vi "Dashboard Main.vi"() -> ()   [LabVIEW 2017]
uses:
  <vilib>/Utility/miscctls.llb/LVRowAndColumnTypeDef.ctl
  <vilib>/event_ctls.llb/eventvkey.ctl
  <vilib>/Rock Robotics/Network Tables/NT Read Numeric Array.vi
  <vilib>/Rock Robotics/WPI/Dashboard/WPI_DashboardLogging Global.vi
  <vilib>/Rock Robotics/Network Tables/NT Read Boolean.vi
panel:
  in  "Camera Settings Right":T1={"Frame Rate"=30, "Compression"=30, "Size"=1, "DB Camera Config"=FALSE} {"Frame Rate" scale=1.0..30.0; "Compression" scale=100.0..-1.0; "Size" items=["640x480", "320x240", "160x120"]}
  in  "Camera Name Right":string(combo)="No Camera Selection"
  out "Camera Info":cluster{"Mbps LED":bool, "Mbps":dbl, "fps":dbl} {"fps" format="%#.1g"; "Mbps" format="%#.1g"}
  in  "Camera Settings":T1={"Frame Rate"=30, "Compression"=30, "Size"=1, "DB Camera Config"=FALSE} {"Frame Rate" scale=1.0..30.0; "Compression" scale=100.0..-1.0; "Size" items=["640x480", "320x240", "160x120"]}
  in  "TCP":refnum<k5>
  in  "Rec Mode":enum32{"Stop", "Record", "Playback"}(radio)
  out "Robot IP":string
  out "Image Message":string="Timeout in Camera Communications"
  in  "Dashboard Tab":T2(tab)
  in  "Select Auto":string(combo)="Select Autonomous ..."
  out "NT Connection":bool
  out "MotorChart R":cluster{"Numeric":dbl, "Numeric":dbl}(graph)
  out "MotorChart L":cluster{"Numeric":dbl, "Numeric":dbl}(graph)
  out "MotorSliders R":cluster{"MotorSlide1":dbl, "MotorSlide2":dbl} {"MotorSlide2" scale=-1.0..1.0 scale format="%#_2e"; "MotorSlide1" scale=-1.0..1.0 scale format="%#_2e"}
  out "MotorSliders L":cluster{"MotorSlide1":dbl, "MotorSlide2":dbl} {"MotorSlide2" scale=-1.0..1.0 scale format="%#_2e"; "MotorSlide1" scale=-1.0..1.0 scale format="%#_2e"}
  out "Gyro":dbl(knob) scale=0.0..360.0
  out "JS1 Z":dbl(slide) scale=-1.0..1.0 scale format="%#_2e"
  out "JS1 Graph":cluster{"X":dbl, "Y":dbl}[](graph)
  out "JS1 Buttons":T3
  out "JS2 Z":dbl(slide) scale=-1.0..1.0 scale format="%#_2e"
  out "JS2 Graph":cluster{"X":dbl, "Y":dbl}[](graph)
  out "JS2 Buttons":T3
  out "Mode":T4(ring)=enum."Auto Disabled"
  out "Camera Image Right":T5(plugin-control)
  in  "DB/String 9":string
  in  "DB/String 8":string
  in  "DB/String 7":string
  in  "DB/String 6":string
  in  "DB/String 5":string
  in  "DB/String 4":string
  in  "DB/String 3":string
  in  "DB/String 2":string
  in  "DB/String 1":string
  in  "DB/String 0":string
  in  "DB/Slider 0":dbl(slide) scale=0.0..5.0
  in  "DB/Slider 1":dbl(slide) scale=0.0..5.0
  in  "DB/Slider 2":dbl(slide) scale=0.0..5.0
  in  "DB/Slider 3":dbl(slide) scale=0.0..5.0
  out "DB/LED 3":bool
  out "DB/LED 2":bool
  out "DB/LED 1":bool
  out "DB/LED 0":bool
  in  "DB/Button 3":bool
  in  "DB/Button 2":bool
  in  "DB/Button 1":bool
  in  "DB/Button 0":bool caption="New Name"
  in  "Test Slider":dbl(slide) scale=0.0..100.0 scale format="%#_3g"
  in  "On/Off":bool caption="Solenoid"
  in  "Test Name":u16(ring) items=["Select the test to run..."]
  in  "Test Tree":string(tree)
  in  "Motor":cluster{"Value":dbl, "Enable":bool} {"Value" scale=-1.0..1.0 scale format="%#_3g"}
  out "Progress":T6 {"Test Progress" scale=0.0..100.0}
  in  "Rev/Fwd":cluster{"Forward":bool, "Reverse":bool}
  in  "Test Ring":u16(ring) items=["Monochrome", "Color"]
  out "Cmd Status":string
  in  "Execute Command":bool
  in  "Command Params":string[][](table)
  in  "Command Selection":i32(listbox)
  in  "CheckList":i32(listbox)
  out "Tree":string(tree)
  out "Camera Image":T5(plugin-control)
  out "Background":bool
  in  "Camera Name":string(combo)="No Camera Selection"
  # "HW"
  # "HW"
  # "Joysticks"
  # "Drive Motors"
  # "Front"
  # "Right"
  # "Left"
  # "Back"
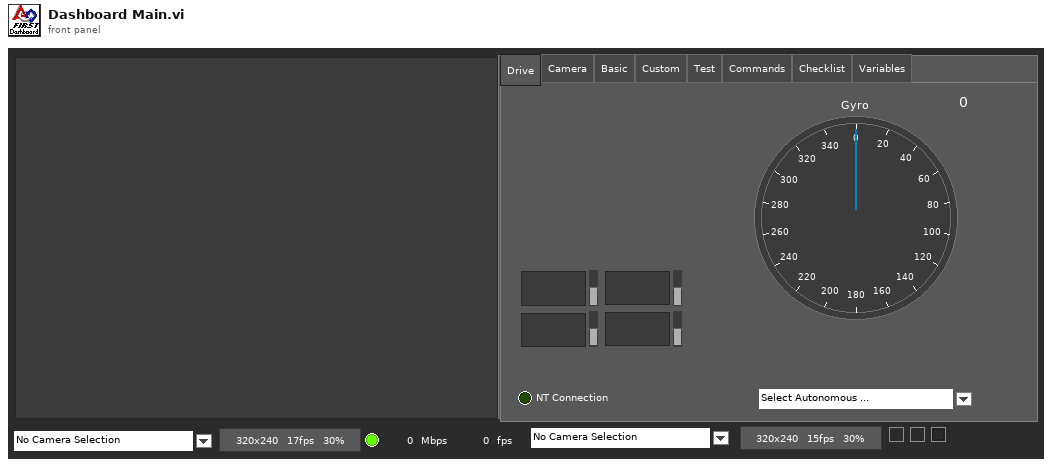
[diagram p1: front panel]
types:
  T1 = cluster{"Frame Rate":i32, "Compression":i32, "Size":u16, "DB Camera Config":bool}
  T2 = enum32{"Drive", "Camera", "Basic", "Custom", "Test", "Commands", "Checklist", "Variables"}
  T3 = cluster{bool, bool, bool, bool, bool, bool, bool, bool, bool, bool, bool, bool}
  T4 = enum8{"Tele-Op Disabled", "Tele-Op Enabled", "Auto Disabled", "Auto Enabled", "Test Disabled", "Test Enabled", "Disconnected", "No Code", "E-Stop"}
  T5 = typedef "IMAQ Image.ctl" = refnum<image>
  T6 = cluster{"Test Progress":u8, "Test Progress Text":string}
  T7 = cluster{"Save Path":path, "Interval (s)":dbl, "Keep":i32}
  T8 = typedef "Image Type" = u32
  T9 = cluster{"IDs":cluster{"RPC field ID":u16, "Unique ID":u16}, "String":string}
  T10 = cluster{"String":string, string, "Saved DB Images Info":cluster{"Save Path":path, "Interval (s)":dbl, "Keep":i32}}
  T11 = cluster{"Camera Image":refnum<vi>, "Dashboard Tab":refnum<vi>, "Background":refnum<vi>, "Rec Mode":refnum<vi>, "Test Slider":refnum<vi>, "On/Off ":refnum<vi>, "Test Ring":refnum<vi>, "Rev/Fwd":refnum<vi>, "Test Name":refnum<vi>, "Motor":refnum<vi>, "Progress":refnum<vi>, "CheckList":refnum<vi>, "Tree":refnum<vi>, "Test Tree":refnum<vi>, "Command Params":refnum<vi>, "Command Selection":refnum<vi>, "Execute Command":refnum<vi>, "Cmd Status":refnum<vi>, "Camera Settings":refnum<vi>, "Camera Name":refnum<vi>, "Camera Info":refnum<vi>, "Camera Settings Right":refnum<vi>, "Camera Name Right":refnum<vi>, "Camera Image Right":refnum<vi>}
  T12 = cluster{"Error Strings":string, "Disable Counts":cluster{u16, u16}, "Rail Faults":cluster{u16, u16, u16}, "Robot IP":string, "DB Mode":u8, "Event Info":cluster{"Name":string, "Type":u8, "Number":u16, "Replay":u8}}
  T13 = cluster{"Storage":cluster{"Disk Free":u64, "RAM Block":u32, "RAM free":u32}, "CPU Utilization":cluster{"CPU % ISR":sgl, "CPU % Time Crit":sgl, "CPU % Timed Str":sgl, "CPU % High":sgl, "CPU % Above":sgl, "CPU % Normal":sgl, "CPU % Low":sgl}, "CAN":cluster{"% Bus Utilization":sgl, "Bus Off Cnt":u32, "TX_FIFO Full Cnt":u32, "Receive Error Cnt":u8, "Transmit Error Cnt":u8}, "HID":cluster{"HID Outputs":u32, "Rumble Low":u16, "Rumble High":u16}[]}
  T14 = cluster{"Status bits":cluster{"Test Mode":bool, "Autonomous":bool, "Enabled":bool, "Code Start":bool, "Brownout":bool, "Reserved 2":bool, "Reserved 3":bool, "E-Stop":bool}, "Code Trace":cluster{"Disabled":bool, "TeleOp":bool, "Auto":bool, "Test":bool}, "Controller Type":enum16{"unknown", "cRIO", "roboRio"}, "Code?":enum16{"unknown", "noCode", "code"}, "Battery V":dbl}
  T15 = cluster{"Control Bits":cluster{"TestMode":bool, "Autonomous":bool, "Enabled":bool, "FMS Present":bool, bool, bool, bool, "E-Stop":bool}, "Team Station ":u8, "Countdown":sgl, "Joystick Values":cluster{"Axes":dbl[], "Buttons":bool[], "POVs":i16[]}[]}
  T16 = cluster{"Axes":dbl[], "Buttons":bool[], "POVs":i16[]}[]
  T17 = cluster{"Axes":dbl[], "Buttons":bool[], "POVs":i16[]}
  T18 = cluster{"Buttons[0]":bool, "Buttons[1]":bool, "Buttons[2]":bool, "Buttons[3]":bool, "Buttons[4]":bool, "Buttons[5]":bool, "Buttons[6]":bool, "Buttons[7]":bool, "Buttons[8]":bool, "Buttons[9]":bool, "Buttons[10]":bool, "Buttons[11]":bool}
  T19 = cluster{"Operation":enum16{"Update", "Clear"}, "Color Box":u32}[]
  T20 = typedef "eventvkey.ctl" = enum16{"ASCII", "Enter", "Return", "Shift", "Ctrl", "Alt", "Cmd", "Opt", "Caps", "NumLock", "Clear", "Break", "Up", "Down", "Left", "Right", "Insert", "Delete", "Home", "End", "PageUp", "PageDown", "Escape", "Help", "Pause", "ScrollLock", "F1", "F2", "F3", "F4", "F5", "F6", "F7", "F8", "F9", "F10", "F11", "F12", "F13", "F14", "F15", "F16", "F17", "F18", "F19", "F20", "F21", "F22", "F23", "F24", "Play", "VolumeUp", "VolumeDown", "Mute", "Two Byte Char"}
  T21 = cluster{"Image Size":bool, "Image Type":bool, "Pixel Value":bool, "ROI Information":bool, "Zoom Factor":bool}
  T22 = cluster{"Operation":enum16{"Update", "Clear"}, "Color Box":u32}
  T23 = typedef "LVRowAndColumnTypeDef.ctl" = cluster{"Row":i32, "Column":i32}
  T24 = cluster{"Shift":bool, "Ctrl":bool, "Alt":bool, "Cmd":bool, "Opt":bool}
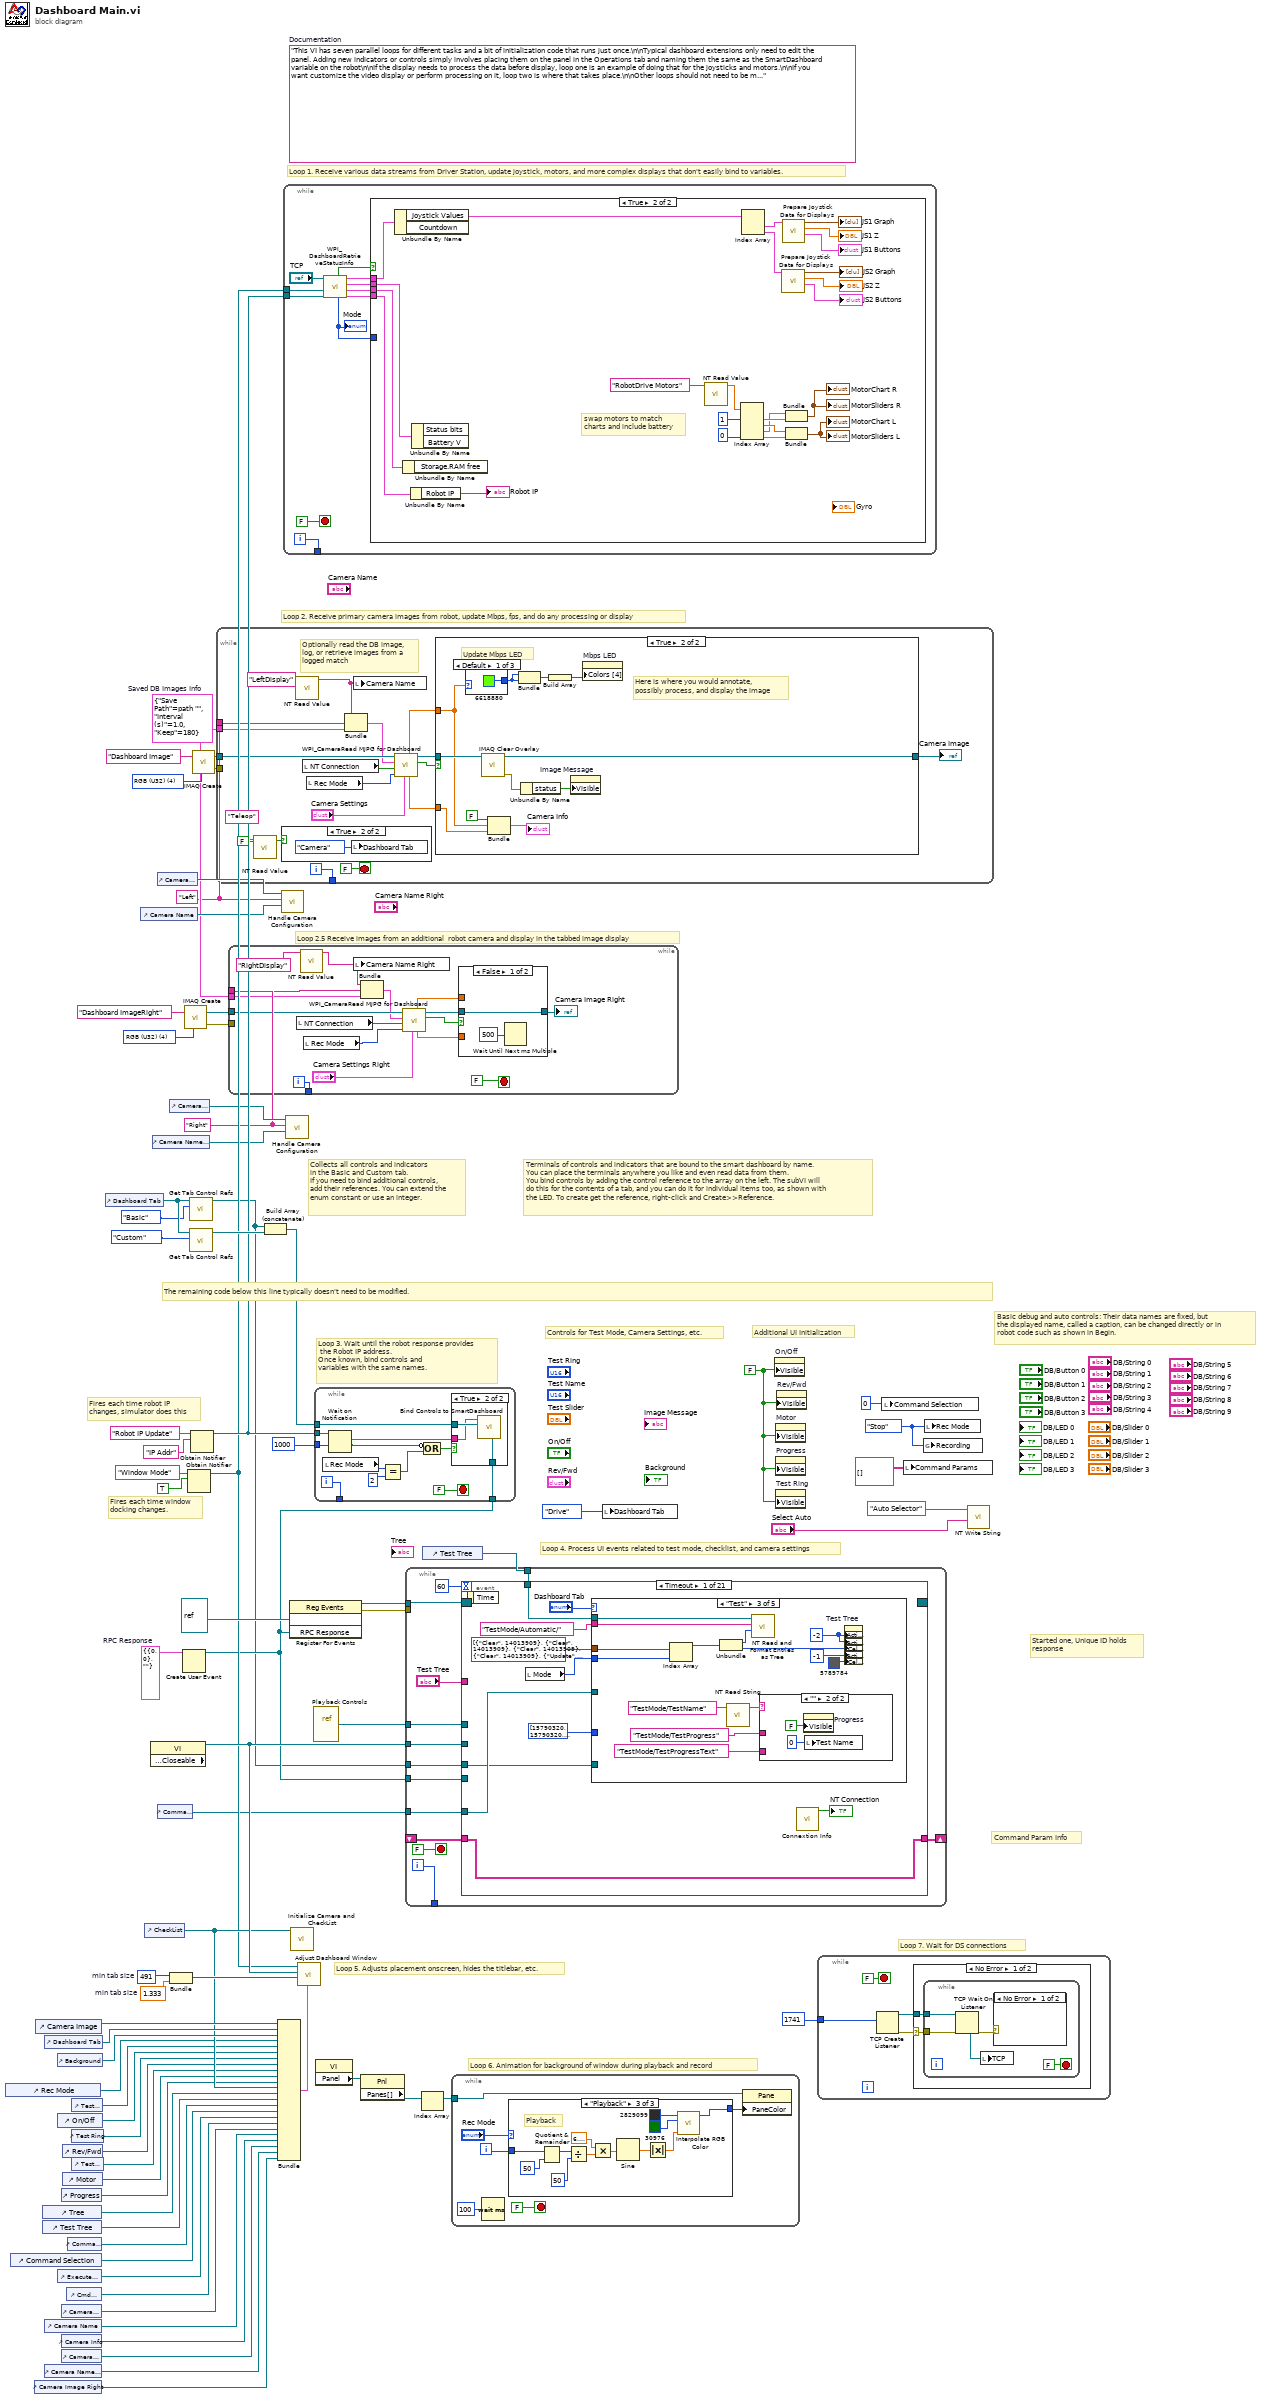
[diagram p0: block diagram]
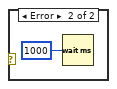
[diagram p3: hidden frame]
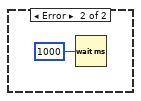
[diagram p4: hidden frame]
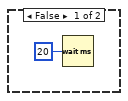
[diagram p5: hidden frame]
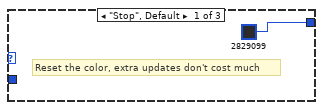
[diagram p6: hidden frame]
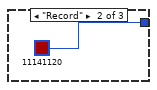
[diagram p7: hidden frame]
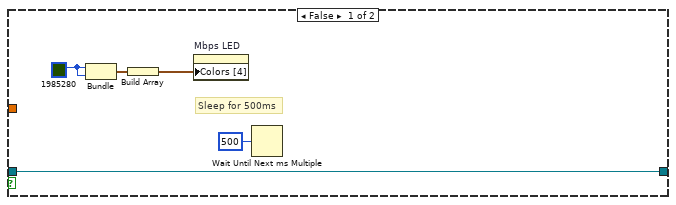
[diagram p10: hidden frame]
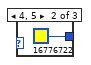
[diagram p11: hidden frame]
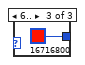
[diagram p12: hidden frame]
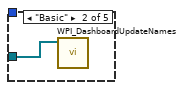
[diagram p14: hidden frame]
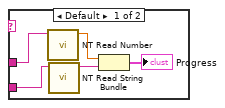
[diagram p15: hidden frame]
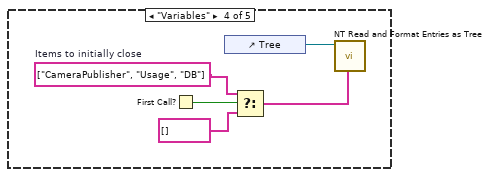
[diagram p16: hidden frame]
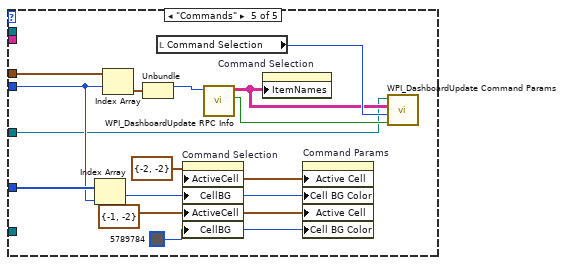
[diagram p17: hidden frame]
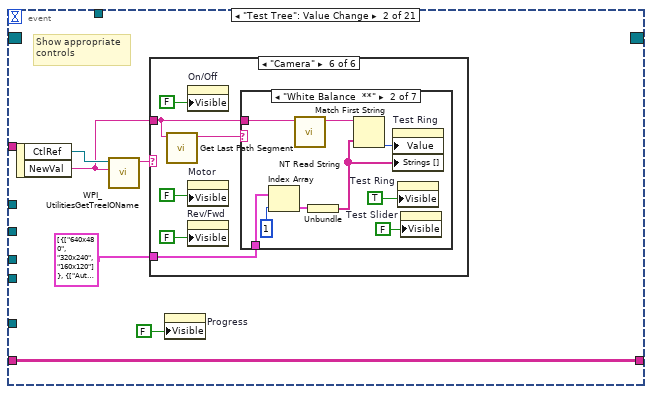
[diagram p18: hidden frame]
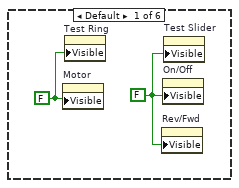
[diagram p19: hidden frame]
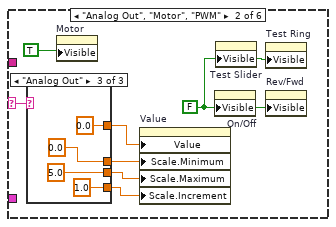
[diagram p20: hidden frame]
diagram:
  w3 = T7 {"Save Path"=path "", "Interval (s)"=1.0, "Keep"=180}  # Saved DB Images Info
  w2 = "Right"
  w1 = "Left"
  w13 = T8 4 items=["Grayscale (U8)", "Grayscale (I16)", "Grayscale (SGL)", "Complex (CSG)", "RGB (U32)", "HSL (U32)", "RGB (U64)"] ("Image Type")
  w29 = T9 {"IDs"={"RPC field ID"=0, "Unique ID"=0}, "String"=""}  # RPC Response
  w52 = 491  # min tab size
  w51 = 1.333  # min tab size
  w59 = enum32{"Stop", "Record", "Playback"}."Stop" ("Rec Mode")
  w36 = FALSE ("Visible")
  (unwired) "This VI has seven parallel loops for different tasks and a bit of initialization code that runs just once.\n\nTypical dashboard extensions only need to edit the panel. Adding new indicators or controls simply involves placing them on the panel in the Operations tab and naming them the same as the SmartDashboard variable on the robot\n\nIf the display needs to process the data before display, loop one is an example of doing that for the joysticks and motors.\n\nIf you want customize the video display or perform processing on it, loop two is where that takes place.\n\nOther loops should not need to be modified. They are pretty standard, and document the task they perform."  # Documentation
  w76 = T8 4 items=["Grayscale (U8)", "Grayscale (I16)", "Grayscale (SGL)", "Complex (CSG)", "RGB (U32)", "HSL (U32)", "RGB (U64)"] ("Image Type")
  # "Loop 2.5 Receive images from an additional  robot camera and display in the tabbed image display"
  # "Command Param Info"
  # "Started one, Unique ID holds\nresponse"
  # "Loop 7. Wait for DS connections"
  # "Basic debug and auto controls: Their data names are fixed, but\nthe displayed name, called a caption, can be changed directly or in\nrobot code such as shown in Begin."
  # "Controls for Test Mode, Camera Settings, etc."
  # "Additional UI Initialization"
  # "Loop 6. Animation for background of window during playback and record"
  # "Fires each time robot IP\nchanges, simulator does this"
  # "Fires each time window\ndocking changes."
  # "Collects all controls and indicators\nin the Basic and Custom tab.\nIf you need to bind additional controls,\nadd their references. You can extend the\nenum constant or use an integer."
  # "The remaining code below this line typically doesn't need to be modified."
  # "Loop 4. Process UI events related to test mode, checklist, and camera settings"
  # "Terminals of controls and indicators that are bound to the smart dashboard by name.\nYou can place the terminals anywhere you like and even read data from them.\nYou bind controls by adding the control reference to the array on the left. The subVI will\ndo this for the contents of a tab, and you can do it for individual items too, as shown with\nthe LED. To create get the reference, right-click and Create>>Reference."
  # "Loop 3. Wait until the robot response provides\n the Robot IP address.\nOnce known, bind controls and\nvariables with the same names."
  # "Loop 5. Adjusts placement onscreen, hides the titlebar, etc."
  # "Loop 1. Receive various data streams from Driver Station, update joystick, motors, and more complex displays that don't easily bind to variables."
  # "Loop 2. Receive primary camera images from robot, update Mbps, fps, and do any processing or display"
  n1 = control-ref of="Rec Mode"() -> (w42:refnum<vi>)
  n2 = control-ref of="Command Selection"() -> (w28:refnum<vi>)
  n3 = control-ref of="Camera Image Right"() -> (w6:refnum<vi>)
  n4 = control-ref of="Camera Image"() -> (w54:refnum<vi>)
  n5 = control-ref of="Tree"() -> (w46:refnum<vi>)
  n6 = control-ref of="Test Tree"() -> (w45:refnum<vi>)
  n7 = control-ref of="Dashboard Tab"() -> (w53:refnum<vi>)
  n8 = control-ref of="Camera Name"() -> (w19:refnum<vi>)
  n9 = control-ref of="Camera Name Right"() -> (w7:refnum<vi>)
  n10 = control-ref of="Execute Command"() -> (w30:refnum<vi>)
  n11 = control-ref of="Background"() -> (w49:refnum<vi>)
  n12 = control-ref of="On/Off"() -> (w40:refnum<vi>)
  n13 = control-ref of="Progress"() -> (w37:refnum<vi>)
  n14 = control-ref of="Camera Settings"() -> (w20:refnum<vi>)
  n15 = control-ref of="Camera Info"() -> (w18:refnum<vi>)
  n16 = control-ref of="Camera Settings Right"() -> (w8:refnum<vi>)
  n17 = control-ref of="Rev/Fwd"() -> (w38:refnum<vi>)
  n18 = control-ref of="Motor"() -> (w43:refnum<vi>)
  n19 = control-ref of="Cmd Status"() -> (w24:refnum<vi>)
  n20 = control-ref of="Command Params"() -> (w31:refnum<vi>)
  n21 = control-ref of="Test Slider"() -> (w41:refnum<vi>)
  n22 = control-ref of="Test Ring"() -> (w39:refnum<vi>)
  n23 = control-ref of="Test Name"() -> (w44:refnum<vi>)
  n24 = control-ref of="Dashboard Tab"() -> (w57:refnum<vi>)
  n25 = control-ref of="Camera Name"() -> (w21:refnum<vi>)
  n26 = control-ref of="CheckList"() -> (w47:refnum<vi>)
  n27 = property class="VI" props=["Front Panel.Closeable"]() -> (reference out=w58:refnum<vi>)  [unwired: 2 in, 2 out]
  n28 = control-ref of="Camera Name Right"() -> (w9:refnum<vi>)
  n29 = control-ref of="Camera Settings"() -> (w22:refnum<vi>)
  n30 = control-ref of="Command Params"() -> (w23:refnum<vi>)
  n31 = control-ref of="Camera Settings Right"() -> (w10:refnum<vi>)
  n32 = Bundle("min tab size"=w52, "min tab size"=w51) -> (w50:cluster{"min tab size":i32, "min tab size":dbl})  [unwired: 1 in]
  n33 = Create User Event(user event datatype=w29) -> (user event=w25:refnum<user-event>)  [unwired: 1 in, 1 out]
  n34 = call "IMAQ Create"("Image Name"="Dashboard ImageRight", "Image Type"=w13) -> ("New Image"=w12:T5, "error out"=w11:errorcluster)  [unwired: 2 in, 1 out]
  n35 = Obtain Notifier(name (unnamed)="Window Mode", notification data type=TRUE) -> (notifier out=w34:refnum<notifier>)  [unwired: 2 in, 2 out]
  n36 = call <vilib>:"Get Tab Control Refs.vi"("Page Index"=T2."Basic" ("Dashboard Tab"), "TabControl in"=w57) -> ("ControlsOnPage"=w17:refnum<vi>[])  [unwired: 9 in]
  n37 = call <vilib>:"Get Tab Control Refs.vi"("Page Index"=T2."Custom" ("Dashboard Tab"), "TabControl in"=w57) -> ("ControlsOnPage"=w56:refnum<vi>[])  [unwired: 9 in]
  n38 = Obtain Notifier(name (unnamed)="Robot IP Update", notification data type="IP Addr" ("name (unnamed)")) -> (notifier out=w35:refnum<notifier>)  [unwired: 2 in, 2 out]
  n39 = call "IMAQ Create"("Image Name"="Dashboard Image", "Image Type"=w76) -> ("New Image"=w74:T5, "error out"=w73:errorcluster)  [unwired: 2 in, 1 out]
  n40 = while {
    tunnel: w74 -> [w93]
    tunnel: w73 -> [_]
    tunnel: [w94] -> _
    tunnel: w3 -> [w84]
    tunnel: w1 -> [w82]
    i -> [w94]
    stop <- FALSE stop-if-true
    # "Optionally read the DB image,\nlog, or retrieve images from a\nlogged match"
    n41 = call-poly <vilib>:"NT Read Value.vi"("Default Value"=FALSE, "Name"="Teleop") -> ("Boolean"=w79:bool)  [unwired: 8 in, 1 out]
    n42 = case shown="True" w79 {
      frame False {
      }
      frame True {
        n43 = local write "Dashboard Tab"(T2."Camera" ("Dashboard Tab")) -> ()
      }
    }
    n44 = call-poly <vilib>:"NT Read Value.vi"("Name"="LeftDisplay") -> ("String"=w81:string)  [unwired: 9 in, 1 out]
    n45 = local read "NT Connection"() -> (w85:bool)
    n46 = local read "Rec Mode"() -> (w89:enum32{"Stop", "Record", "Playback"})
    n47 = Bundle("String"=w81, w82, "Saved DB Images Info"=w84) -> (w83:T10)  [unwired: 1 in]
    n48 = local write "Camera Name"(w81) -> ()
    n49 = call <vilib>:"WPI_CameraRead MJPG for Dashboard.vi"("Camera Settings"="Camera Settings", "Rec Mode"=w89, "NT Connection"=w85, "Capture Info"=w83, "Refnum in"=w93) -> ("Active"=w91:bool, "Refnum out"=w92:T5, "FPS"=w90:dbl, "Bandwidth (Mbps)"=w88:dbl)  [unwired: 3 in]
    n50 = case shown="True" w91 {
      tunnel: w92 -> [w97 w108]
      tunnel: w88 -> [_ w105]
      tunnel: w90 -> [_ w106]
      tunnel: [w97 w102] -> w86
      frame False {
        w99 = u32 1985280 ("Color Box")
        # "Sleep for 500ms"
        n51 = Bundle("Color Box"=w99, "Color Box"=w99) -> (w100:cluster{"Color Box":u32, "Color Box":u32})  [unwired: 1 out]
        n52 = Build Array(w100) -> (w98:cluster{"Color Box":u32, "Color Box":u32}[])
        n53 = property on="Mbps LED" class="Bool (strict)"("Colors [4]"=w98) -> ()  [unwired: 2 in, 2 out]
        n54 = Wait Until Next ms Multiple(millisecond multiple=u32 500) -> ()  [unwired: 1 out]
      }
      frame True {
        # "Here is where you would annotate,\npossibly process, and display the image"
        # "Update Mbps LED"
        n55 = case shown="Default" w105 {
          tunnel: [u32 6618880 ("Color Box") u32 16776722 ("Color Box") u32 16716800 ("Color Box")] -> w109
          frame Default {
          }
          frame 4, 5 {
          }
          frame 6.. {
          }
        }
        n56 = call "IMAQ Clear Overlay"("Image"=w108) -> ("error out"=w111:errorcluster, "Image Out"=w102:T5)  [unwired: 2 in, 7 out]
        n57 = Bundle(FALSE, "Bandwidth (Mbps)"=w105, "FPS"=w106) -> (→"Camera Info":cluster{bool, "Bandwidth (Mbps)":dbl, "FPS":dbl})  [unwired: 1 in]
        n58 = Bundle("Color Box"=w109, "Color Box"=w109) -> (w110:cluster{"Color Box":u32, "Color Box":u32})  [unwired: 1 out]
        n59 = Unbundle By Name(w111) -> ("status"=w112:bool)
        n60 = Build Array(w110) -> (w107:cluster{"Color Box":u32, "Color Box":u32}[])
        n61 = property on="Image Message" class="Str"("Visible"=w112) -> ()  [unwired: 2 in, 2 out]
        n62 = property on="Mbps LED" class="Bool (strict)"("Colors [4]"=w107) -> ()  [unwired: 2 in, 2 out]
      }
    }
    "Camera Image" <- w86
  }
  n63 = while {
    tunnel: w12 -> [w131]
    tunnel: w11 -> [_]
    tunnel: [w126] -> _
    tunnel: w3 -> [w120]
    tunnel: w2 -> [w119]
    i -> [w126]
    stop <- FALSE stop-if-true
    n64 = local read "NT Connection"() -> (w121:bool)
    n65 = call-poly <vilib>:"NT Read Value.vi"("Name"="RightDisplay") -> ("String"=w116:string)  [unwired: 9 in, 1 out]
    n66 = local read "Rec Mode"() -> (w130:enum32{"Stop", "Record", "Playback"})
    n67 = local write "Camera Name Right"(w116) -> ()
    n68 = Bundle("String"=w116, w119, "Saved DB Images Info"=w120) -> (w117:T10)  [unwired: 1 in]
    n69 = call <vilib>:"WPI_CameraRead MJPG for Dashboard.vi"("Camera Settings"="Camera Settings Right", "Rec Mode"=w130, "NT Connection"=w121, "Capture Info"=w117, "Refnum in"=w131) -> ("Active"=w125:bool, "Refnum out"=w128:T5, "FPS"=w123:dbl, "Bandwidth (Mbps)"=w124:dbl)  [unwired: 3 in]
    n70 = case shown="False" w125 {
      tunnel: w128 -> [w132 w134]
      tunnel: w124 -> [_ _]
      tunnel: w123 -> [_ _]
      tunnel: [w132 w134] -> w122
      frame False {
        n71 = Wait Until Next ms Multiple(millisecond multiple=u32 500) -> ()  [unwired: 1 out]
      }
      frame True {
      }
    }
    "Camera Image Right" <- w122
  }
  n72 = Build Array (concatenate)(w17, w56) -> (w55:refnum<vi>[])
  n73 = Bundle("Camera Image"=w54, "Dashboard Tab"=w53, "Background"=w49, "Rec Mode"=w42, "Test Slider"=w41, "On/Off"=w40, "Test Ring"=w39, "Rev/Fwd"=w38, "Test Name"=w44, "Motor"=w43, "Progress"=w37, "CheckList"=w47, "Tree"=w46, "Test Tree"=w45, "Command Params"=w31, "Command Selection"=w28, "Execute Command"=w30, "Cmd Status"=w24, "Camera Settings"=w20, "Camera Name"=w19, "Camera Info"=w18, "Camera Settings Right"=w8, "Camera Name Right"=w7, "Camera Image Right"=w6) -> (w48:T11)  [unwired: 1 in]
  n74 = call "Handle Camera Configuration.vi"("CameraNameRef"=w21, "Display Name"=w1, "ClusterRef"=w22) -> ()  [unwired: 9 in]
  n75 = while {
    tunnel: [w144] -> _
    tunnel: w35 -> [w138]
    tunnel: w34 -> [w135]
    i -> [w144]
    stop <- FALSE stop-if-true
    n76 = call <vilib>:"WPI_DashboardRetrieveStatusInfo.vi"("Binding Refnum"=w138, "Window Mode Notifier"=w135, "TCP Cnx"="TCP") -> ("Power and Errors"=w139:T12, "Robot Metrics"=w142:T13, "Status Info"=w143:T14, "Control Info"=w140:T15, "Robot Mode"=w137:T4, "Process?"=w141:bool)  [unwired: 3 in]
    "Mode" <- w137
    n77 = case shown="True" w141 {
      tunnel: w143 -> [_ w170]
      tunnel: w142 -> [_ w169]
      tunnel: w140 -> [_ w168]
      tunnel: w139 -> [_ w167]
      tunnel: w137 -> [_ _]
      frame False {
        n78 = Wait (ms)(milliseconds to wait=u32 20) -> ()  [unwired: 1 out]
      }
      frame True {
        # "swap motors to match\ncharts and include battery"
        n79 = Unbundle By Name(w168) -> ("Joystick Values"=w158:T16)  [unwired: 1 out]
        n80 = Unbundle By Name(w169) -> ()  [unwired: 1 out]
        n81 = Unbundle By Name(w167) -> ("Robot IP"=→"Robot IP":string)
        n82 = Unbundle By Name(w170) -> ()  [unwired: 2 out]
        n83 = call-poly <vilib>:"NT Read Value.vi"("Name"="RobotDrive Motors") -> ("Numeric Array"=w148:dbl[])  [unwired: 9 in, 1 out]
        n84 = Index Array(array=w148, index #1=1, index #4=0) -> (element #1=w162:dbl, element #2=w163:dbl, element #3=w161:dbl, element #4=w166:dbl)  [unwired: 2 in]
        n85 = Index Array(array=w158) -> (element #1=w157:T17, element #2=w153:T17)  [unwired: 2 in]
        n86 = call "Prepare Joystick Data for Displays.vi"("Joystick Values"=w153) -> ("Buttons"=→"JS2 Buttons":T18, "Z Axis"=→"JS2 Z":dbl, "Cartesian Data"=→"JS2 Graph":cluster{"X axis":dbl, "X axis":dbl}[])  [unwired: 8 in]
        n87 = call "Prepare Joystick Data for Displays.vi"("Joystick Values"=w157) -> ("Buttons"=→"JS1 Buttons":T18, "Z Axis"=→"JS1 Z":dbl, "Cartesian Data"=→"JS1 Graph":cluster{"X axis":dbl, "X axis":dbl}[])  [unwired: 8 in]
        n88 = Bundle("Numeric"=w161, "Numeric"=w162) -> (→"MotorChart R" →"MotorSliders R":cluster{"Numeric":dbl, "Numeric":dbl})  [unwired: 1 in]
        n89 = Bundle("Numeric"=w163, "Numeric"=w166) -> (→"MotorChart L" →"MotorSliders L":cluster{"Numeric":dbl, "Numeric":dbl})  [unwired: 1 in]
      }
    }
  }
  n90 = call "Handle Camera Configuration.vi"("CameraNameRef"=w9, "Display Name"=w2, "ClusterRef"=w10) -> ()  [unwired: 9 in]
  n91 = register-events(refnum<vi> refnum, w25) -> (reference out=w63:refnum<event-registration>, error out=w62:errorcluster)  [unwired: 2 in]
  n92 = call "Initialize Camera and CheckList.vi"("ListBox in"=w47) -> ()  [unwired: 11 in]
  n93 = call "Adjust Dashboard Window.vi"("Sizing Refnums"=w48, "Size Constraints"=w50, "VI"=w58, "WIn Mode"=w34) -> ()  [unwired: 8 in]
  n94 = vi-ref "Playback Controls.vi"() -> (w64:refnum<vi>)
  n95 = while {
    tunnel: w55 -> [w182]
    tunnel: w35 -> [w180]
    tunnel: [w178] -> _
    tunnel: u32 1000 ("milliseconds to wait") -> [w177]
    tunnel: w25 -> [w171]
    i -> [w178]
    stop <- FALSE stop-if-true
    n96 = local read "Rec Mode"() -> (w173:enum32{"Stop", "Record", "Playback"})
    n97 = Wait on Notification(notifier=w180, timeout in ms (-1)=w177) -> (notification=w179:string, timed out?=w175:bool)  [unwired: 2 in, 2 out]
    n98 = Equal?(x=w173, y=u16 2 ("Rec Mode")) -> (x = y?=w174:bool)
    n99 = Compound Arithmetic op=OR(invert w175, w174) -> (w176:bool)
    n100 = case shown="True" w176 {
      tunnel: w182 -> [_ w185]
      tunnel: w179 -> [_ w184]
      tunnel: w171 -> [_ w183]
      frame False {
      }
      frame True {
        n101 = call <vilib>:"Bind Controls to SmartDashboard.vi"("RPC ref"=w183, "Bound Control Refs"=w185, "Server IP Address"=w184) -> ()  [unwired: 9 in]
      }
    }
  }
  n102 = property class="VI"() -> ("Panel"=w66:refnum<vi>)  [unwired: 2 in, 2 out]
  n103 = property class="Pnl"(reference=w66) -> ("Panes[]"=w67:refnum<vi>[])  [unwired: 1 in, 2 out]
  n104 = Index Array(array=w67) -> (element=w65:refnum<vi>)  [unwired: 1 in]
  n105 = control-ref of="Test Tree"() -> (w68:refnum<vi>)
  n106 = while {
    tunnel: [w195] -> _
    tunnel: w68 -> [w194]
    tunnel: w64 -> [w193]
    tunnel: w63 -> [w192]
    tunnel: w62 -> [_]
    tunnel: w58 -> [w191]
    tunnel: w25 -> [w190]
    tunnel: w23 -> [w189]
    shift-right: [w188] -> _
    shift-left: _ -> [w187]
    tunnel: w17 -> [w186]
    i -> [w195]
    stop <- FALSE stop-if-true
    n107 = event shown="[0] Timeout" {
      selector: w192 -> [_ _ _ _ _ _ _ _ _ _ _ _ _ _ _ _ _ _ _ _ _]
      dyn-events: [_ _ _ _ _ _ _ _ _ _ _ _ _ _ _ _ w455 _ _ _ _] -> _
      timeout: u32 60 ("milliseconds to wait") -> [_ _ _ _ _ _ _ _ _ _ _ _ _ _ _ _ _ _ _ _ _]
      tunnel: w194 -> [w207 _ _ _ _ _ _ _ _ _ _ _ _ _ _ _ _ _ _ _ _]
      tunnel: "Test Tree" -> [_ _ _ _ _ _ _ _ _ _ _ w422 w430 w432 w436 w444 _ _ _ _ _]
      tunnel: w193 -> [_ _ _ _ _ _ _ _ _ _ _ _ _ _ _ _ w457 _ w475 _ _]
      tunnel: w191 -> [_ _ _ _ _ _ _ _ _ _ _ _ _ _ _ _ w453 _ _ _ _]
      tunnel: w190 -> [_ _ _ _ _ _ _ _ _ _ _ _ _ _ _ _ w451 _ _ _ _]
      tunnel: w189 -> [w202 _ _ _ _ _ w373 _ _ _ _ _ _ _ _ _ _ _ _ _ _]
      tunnel: [w201 w250 w352 w357 w366 w370 w371 w380 w390 w397 w409 w421 w428 w431 w435 w443 w450 w470 w472 w476 w489] -> w188
      tunnel: w187 -> [w201 w250 w352 w357 w366 w370 w371 _ _ w397 w409 w421 w428 w431 w435 w443 w450 w470 w472 w476 w489]
      tunnel: w186 -> [w199 _ _ _ _ _ _ _ _ _ _ _ _ _ _ _ _ _ _ _ _]
      event Timeout {
        n108 = event-data() -> ()  [unwired: 1 in, 1 out]
        n109 = local read "Mode"() -> (w204:T4)
        n110 = case shown="\"Test\"" "Dashboard Tab" {
          tunnel: w207 -> [_ _ w223 _ _]
          tunnel: "TestMode/Automatic/" ("Name Pattern") -> [_ _ w222 _ _]
          tunnel: T19 [{"Operation"=enum."Clear", "Color Box"=14013909}, {"Operation"=enum."Clear", "Color Box"=14013909}, {"Operation"=enum."Clear", "Color Box"=14013909}, {"Operation"=enum."Clear", "Color Box"=14013909}, {"Operation"=enum."Update", "Color Box"=14013909}, {"Operation"=enum."Update", "Color Box"=16777215}, {"Operation"=enum."Clear", "Color Box"=14013909}, {"Operation"=enum."Clear", "Color Box"=14013909}, {"Operation"=enum."Clear", "Color Box"=14013909}] -> [_ _ w215 _ w243]
          tunnel: w204 -> [_ _ w214 _ w242]
          tunnel: u32[] [15790320, 15790320, 15790320, 15790320, 16777215, 16777215, 15790320, 15790320, 15790320] -> [_ _ _ _ w248]
          tunnel: w202 -> [_ _ _ _ w236]
          tunnel: w199 -> [_ w209 _ _ _]
          frame "Custom", Default {
          }
          frame "Basic" {
            n111 = call <vilib>:"WPI_DashboardUpdateNames.vi"("Controls on Tab"=w209) -> ()  [unwired: 11 in]
          }
          frame "Test" {
            w221 = -2 ("Active Item:Row Number")
            n112 = Index Array(array=w215, index=w214) -> (element=w216:T22)
            n113 = Unbundle(w216) -> ("Operation"=w217:enum16{"Update", "Clear"}, "Color Box"=w218:u32)
            n114 = call <vilib>:"NT Read String.vi"("Name"="TestMode/TestName") -> ("String"=w212:string)  [unwired: 9 in, 1 out]
            n115 = call <vilib>:"NT Read and Format Entries as Tree.vi"("Operation"=w217, "Name Pattern"=w222, "Tree Refnum"=w223) -> ()  [unwired: 7 in, 2 out]
            n116 = case shown="\"\"" w212 {
              tunnel: "TestMode/TestProgress" ("Name") -> [w225 _]
              tunnel: "TestMode/TestProgressText" ("Name") -> [w224 _]
              frame Default {
                n117 = call <vilib>:"NT Read Number.vi"("Name"=w225) -> ("Numeric"=w226:dbl)  [unwired: 9 in, 1 out]
                n118 = call <vilib>:"NT Read String.vi"("Name"=w224) -> ("String"=w227:string)  [unwired: 9 in, 1 out]
                n119 = Bundle("Numeric"=w226, "String"=w227) -> (→"Progress":cluster{"Numeric":dbl, "String":string})  [unwired: 1 in]
              }
              frame "" {
                n120 = property on="Progress" class="Clust (strict)"("Visible"=FALSE) -> ()  [unwired: 2 in, 2 out]
                n121 = local write "Test Name"(u16 0) -> ()
              }
            }
            n122 = property on="Test Tree" class="Tree (strict)"("Active Item Row Number"=w221, "ActiveColNum"=w221, "CellBG"=w218, "Active Item Row Number"=-1 ("Active Item:Row Number"), "CellBG"=u32 5789784 ("Color Box")) -> ()  [unwired: 2 in, 2 out]
          }
          frame "Variables" {
            w233 = string[] ["CameraPublisher", "Usage", "DB"]  # Items to initially close
            n123 = First Call?() -> (First Call?: T/F=w234:bool)
            n124 = control-ref of="Tree"() -> (w235:refnum<vi>)
            n125 = Select(t=w233, s=w234, f=string[] []) -> (s? t:f=w231:string[])
            n126 = call <vilib>:"NT Read and Format Entries as Tree.vi"("Tags to  Close"=w231, "Tree Refnum"=w235) -> ()  [unwired: 8 in, 2 out]
          }
          frame "Commands" {
            w244 = u32 5789784 ("Color Box")
            w245 = T23 {"Row"=-1, "Column"=-2} ("Active Cell:Active Cell")
            w247 = T23 {"Row"=-2, "Column"=-2} ("Active Cell:Active Cell")
            n127 = Index Array(array=w248, index=w242) -> (element=w246:u32)
            n128 = Index Array(array=w243, index=w242) -> (element=w241:T22)
            n129 = Unbundle(w241) -> ("Operation"=w240:enum16{"Update", "Clear"})  [unwired: 1 out]
            n130 = local read "Command Selection"() -> (w239:i32)
            n131 = property on="Command Selection" class="MCListbox (strict)"("ActiveCell"=w247, "CellBG"=w246, "ActiveCell"=w245, "CellBG"=w244) -> ()  [unwired: 2 in, 2 out]
            n132 = call <vilib>:"WPI_DashboardUpdate RPC Info.vi"("Operation"=w240) -> ("update"=w238:bool, "commands"=w237:string[][])  [unwired: 9 in]
            n133 = property on="Command Selection" class="MCListbox (strict)"("ItemNames"=w237) -> ()  [unwired: 2 in, 2 out]
            n134 = property on="Command Params" class="Tbl (strict)"("Active Cell"=w247, "Cell BG Color"=w246, "Active Cell"=w245, "Cell BG Color"=w244) -> ()  [unwired: 2 in, 2 out]
            n135 = call <vilib>:"WPI_DashboardUpdate Command Params.vi"("Update"=w238, "NewVal"=w239, "Commands"=w237, "Param Tbl"=w236) -> ()  [unwired: 7 in, 1 out]
          }
        }
        n136 = call <vilib>:"Connextion Info.vi"() -> ("Connected"=→"NT Connection":bool)  [unwired: 10 in, 1 out]
      }
      event "Test Tree": Value Change {
        # "Show appropriate\ncontrols"
        n137 = event-data() -> ("CtlRef"=w253:refnum<vi>, "NewVal"=w251:string)  [unwired: 1 in]
        n138 = call <vilib>:"WPI_UtilitiesGetTreeIOName.vi"("NewVal"=w251, "TreeControl in"=w253) -> ("I/O Name"=w254:string)  [unwired: 9 in]
        n139 = case shown="\"Camera\"" w254 {
          selector: w254 -> [_ w261 _ w283 w292 _]
          tunnel: w251 -> [_ _ w280 w282 _ w299]
          tunnel: cluster{string[]}[] [{["640x480", "320x240", "160x120"]}, {["Auto", "Fixed indoor", "Fixed outdoor 1", "Fixed outdoor 2", "Fixed fluorescent 1", "Fixed fluorescent 2", "Hold current"]}, {["Auto", "Flicker-free 50 Hz", "Flicker-free 60 Hz", "Hold current"]}, {["None", "Prioritize frame rate", "Prioritize image quality"]}, {["Monochrome", "Color"]}] -> [_ _ _ _ _ w298]
          frame Default {
            w256 = FALSE ("Visible")
            w255 = FALSE ("Visible")
            n140 = property on="Motor" class="Clust (strict)"("Visible"=w255) -> ()  [unwired: 2 in, 2 out]
            n141 = property on="Test Ring" class="Ring (strict)"("Visible"=w255) -> ()  [unwired: 2 in, 2 out]
            n142 = property on="Rev/Fwd" class="Clust (strict)"("Visible"=w256) -> ()  [unwired: 2 in, 2 out]
            n143 = property on="On/Off" class="Bool (strict)"("Visible"=w256) -> ()  [unwired: 2 in, 2 out]
            n144 = property on="Test Slider" class="Slide (strict)"("Visible"=w256) -> ()  [unwired: 2 in, 2 out]
          }
          frame "Analog Out", "Motor", "PWM" {
            w262 = FALSE ("Visible")
            n145 = case shown="\"Analog Out\"" w261 {
              tunnel: [1.0 ("Value") -1.0 ("Value") 0.0 ("Value")] -> w260
              tunnel: [255.0 ("Value") 1.0 ("Value") 5.0 ("Value")] -> w259
              tunnel: [128.0 ("Value") 0.0 ("Value") 0.0 ("Value")] -> w258
              tunnel: [64.0 ("Value") 0.5 ("Value") 1.0 ("Value")] -> w257
              frame "PWM" {
              }
              frame "Motor", Default {
              }
              frame "Analog Out" {
              }
            }
            n146 = property on="Motor" class="Clust (strict)"("Visible"=TRUE) -> ()  [unwired: 2 in, 2 out]
            n147 = property on="Value" class="Slide (strict)"("Value"=w258, "Scale.Minimum"=w260, "Scale.Maximum"=w259, "Scale.Increment"=w257) -> ()  [unwired: 2 in, 2 out]
            n148 = property on="On/Off" class="Bool (strict)"("Visible"=w262) -> ()  [unwired: 2 in, 2 out]
            n149 = property on="Test Slider" class="Slide (strict)"("Visible"=w262) -> ()  [unwired: 2 in, 2 out]
            n150 = property on="Test Ring" class="Ring (strict)"("Visible"=w262) -> ()  [unwired: 2 in, 2 out]
            n151 = property on="Rev/Fwd" class="Clust (strict)"("Visible"=w262) -> ()  [unwired: 2 in, 2 out]
          }
          frame "Servo" {
            w278 = FALSE ("Visible")
            n152 = call <vilib>:"NT Read Number.vi"("Name"=w280) -> ("Numeric"=w279:dbl)  [unwired: 9 in, 1 out]
            n153 = property on="Test Slider" class="Slide (strict)"("Visible"=TRUE, "Scale.Maximum"=170.0 ("Scale.Range:Maximum")) -> ()  [unwired: 2 in, 2 out]
            n154 = local write "Test Slider"(w279) -> ()
            n155 = property on="Motor" class="Clust (strict)"("Visible"=w278) -> ()  [unwired: 2 in, 2 out]
            n156 = property on="Rev/Fwd" class="Clust (strict)"("Visible"=w278) -> ()  [unwired: 2 in, 2 out]
            n157 = property on="On/Off" class="Bool (strict)"("Visible"=w278) -> ()  [unwired: 2 in, 2 out]
            n158 = property on="Test Ring" class="Ring (strict)"("Visible"=w278) -> ()  [unwired: 2 in, 2 out]
          }
          frame "Relay", "Solenoid" {
            w281 = FALSE ("Visible")
            n159 = property on="Motor" class="Clust (strict)"("Visible"=w281) -> ()  [unwired: 2 in, 2 out]
            n160 = property on="Test Slider" class="Slide (strict)"("Visible"=w281) -> ()  [unwired: 2 in, 2 out]
            n161 = Search and Replace String(input string=w282, search string="/Value  **", replace string="/Direction") -> (result string=w288:string)  [unwired: 5 in, 3 out]
            n162 = property on="Test Ring" class="Ring (strict)"("Visible"=w281) -> ()  [unwired: 2 in, 2 out]
            n163 = call <vilib>:"NT Read String.vi"("Name"=w288) -> ("String"=w286:string)  [unwired: 9 in, 1 out]
            n164 = Equal?(x="Both directions", y=w286) -> (x = y?=w284:bool)
            n165 = Not(x=w284) -> (.not. x?=w285:bool)
            n166 = property on="Rev/Fwd" class="Clust (strict)"("Visible"=w284) -> ()  [unwired: 2 in, 2 out]
            n167 = property on="On/Off" class="Bool (strict)"("Visible"=w285, "Caption.Text"=w283) -> ()  [unwired: 2 in, 2 out]
          }
          frame "Compressor", "Digital Out" {
            w291 = FALSE ("Visible")
            # "Get direction and finish"
            n168 = property on="Motor" class="Clust (strict)"("Visible"=w291) -> ()  [unwired: 2 in, 2 out]
            n169 = property on="Test Slider" class="Slide (strict)"("Visible"=w291) -> ()  [unwired: 2 in, 2 out]
            n170 = property on="Test Ring" class="Ring (strict)"("Visible"=w291) -> ()  [unwired: 2 in, 2 out]
            n171 = property on="On/Off" class="Bool (strict)"("Visible"=TRUE, "Caption.Text"=w292) -> ()  [unwired: 2 in, 2 out]
            n172 = property on="Rev/Fwd" class="Clust (strict)"("Visible"=FALSE) -> ()  [unwired: 2 in, 2 out]
          }
          frame "Camera" {
            n173 = call <vilib>:"Get Last Path Segment.vi"("String in"=w299) -> ("String out"=w300:string)  [unwired: 10 in]
            n174 = property on="On/Off" class="Bool (strict)"("Visible"=FALSE) -> ()  [unwired: 2 in, 2 out]
            n175 = property on="Motor" class="Clust (strict)"("Visible"=FALSE) -> ()  [unwired: 2 in, 2 out]
            n176 = property on="Rev/Fwd" class="Clust (strict)"("Visible"=FALSE) -> ()  [unwired: 2 in, 2 out]
            n177 = case shown="\"White Balance  **\"" w300 {
              tunnel: w299 -> [w306 w315 w324 w333 w342 _ w348]
              tunnel: w298 -> [w304 w312 w321 w330 w339 _ _]
              frame "Size  **" {
                n178 = Index Array(array=w304) -> (element=w303:cluster{string[]})  [unwired: 1 in]
                n179 = call <vilib>:"NT Read String.vi"("Name"=w306) -> ("String"=w305:string)  [unwired: 9 in, 1 out]
                n180 = Unbundle(w303) -> (w301:string[])
                n181 = Match First String(2:w301, 3:w305) -> (0:w302:i32)  [unwired: 1 out]
                n182 = property on="Test Ring" class="Ring (strict)"("Value"=w302, "Strings []"=w301) -> ()  [unwired: 2 in, 2 out]
                n183 = property on="Test Ring" class="Ring (strict)"("Visible"=TRUE) -> ()  [unwired: 2 in, 2 out]
                n184 = property on="Test Slider" class="Slide (strict)"("Visible"=FALSE) -> ()  [unwired: 2 in, 2 out]
              }
              frame "White Balance  **" {
                n185 = Index Array(array=w312, index=1) -> (element=w313:cluster{string[]})
                n186 = call <vilib>:"NT Read String.vi"("Name"=w315) -> ("String"=w314:string)  [unwired: 9 in, 1 out]
                n187 = Unbundle(w313) -> (w310:string[])
                n188 = Match First String(2:w310, 3:w314) -> (0:w309:i32)  [unwired: 1 out]
                n189 = property on="Test Ring" class="Ring (strict)"("Value"=w309, "Strings []"=w310) -> ()  [unwired: 2 in, 2 out]
                n190 = property on="Test Ring" class="Ring (strict)"("Visible"=TRUE) -> ()  [unwired: 2 in, 2 out]
                n191 = property on="Test Slider" class="Slide (strict)"("Visible"=FALSE) -> ()  [unwired: 2 in, 2 out]
              }
              frame "Exposure  **" {
                n192 = Index Array(array=w321, index=2) -> (element=w322:cluster{string[]})
                n193 = call <vilib>:"NT Read String.vi"("Name"=w324) -> ("String"=w323:string)  [unwired: 9 in, 1 out]
                n194 = Unbundle(w322) -> (w318:string[])
                n195 = Match First String(2:w318, 3:w323) -> (0:w319:i32)  [unwired: 1 out]
                n196 = property on="Test Ring" class="Ring (strict)"("Value"=w319, "Strings []"=w318) -> ()  [unwired: 2 in, 2 out]
                n197 = property on="Test Ring" class="Ring (strict)"("Visible"=TRUE) -> ()  [unwired: 2 in, 2 out]
                n198 = property on="Test Slider" class="Slide (strict)"("Visible"=FALSE) -> ()  [unwired: 2 in, 2 out]
              }
              frame "Exposure Priority  **" {
                n199 = Index Array(array=w330, index=3) -> (element=w331:cluster{string[]})
                n200 = call <vilib>:"NT Read String.vi"("Name"=w333) -> ("String"=w332:string)  [unwired: 9 in, 1 out]
                n201 = Unbundle(w331) -> (w327:string[])
                n202 = Match First String(2:w327, 3:w332) -> (0:w328:i32)  [unwired: 1 out]
                n203 = property on="Test Ring" class="Ring (strict)"("Value"=w328, "Strings []"=w327) -> ()  [unwired: 2 in, 2 out]
                n204 = property on="Test Ring" class="Ring (strict)"("Visible"=TRUE) -> ()  [unwired: 2 in, 2 out]
                n205 = property on="Test Slider" class="Slide (strict)"("Visible"=FALSE) -> ()  [unwired: 2 in, 2 out]
              }
              frame "Color Enable  **" {
                n206 = Index Array(array=w339, index=4) -> (element=w340:cluster{string[]})
                n207 = call <vilib>:"NT Read String.vi"("Name"=w342) -> ("String"=w341:string)  [unwired: 9 in, 1 out]
                n208 = Unbundle(w340) -> (w336:string[])
                n209 = Match First String(2:w336, 3:w341) -> (0:w337:i32)  [unwired: 1 out]
                n210 = property on="Test Ring" class="Ring (strict)"("Value"=w337, "Strings []"=w336) -> ()  [unwired: 2 in, 2 out]
                n211 = property on="Test Ring" class="Ring (strict)"("Visible"=TRUE) -> ()  [unwired: 2 in, 2 out]
                n212 = property on="Test Slider" class="Slide (strict)"("Visible"=FALSE) -> ()  [unwired: 2 in, 2 out]
              }
              frame Default {
                n213 = property on="Test Ring" class="Ring (strict)"("Visible"=FALSE) -> ()  [unwired: 2 in, 2 out]
                n214 = property on="Test Slider" class="Slide (strict)"("Visible"=FALSE) -> ()  [unwired: 2 in, 2 out]
              }
              frame "Brightness  **", "Color Level  **", "Compression  **", "FPS  **", "Sharpness  **" {
                n215 = call <vilib>:"NT Read Number.vi"("Name"=w348) -> ("Numeric"=w347:dbl)  [unwired: 9 in, 1 out]
                n216 = local write "Test Slider"(w347) -> ()
                n217 = property on="Test Slider" class="Slide (strict)"("Visible"=TRUE, "Scale.Maximum"=100.0 ("Scale.Range:Maximum")) -> ()  [unwired: 2 in, 2 out]
                n218 = property on="Test Ring" class="Ring (strict)"("Visible"=FALSE) -> ()  [unwired: 2 in, 2 out]
              }
            }
          }
        }
        n219 = property on="Progress" class="Clust (strict)"("Visible"=FALSE) -> ()  [unwired: 2 in, 2 out]
      }
      event "Test Name": Mouse Enter {
        # "Populate the ring with the list of tests"
        n220 = event-data() -> ()  [unwired: 1 in, 1 out]
        n221 = call <vilib>:"NT Read String Array.vi"("Name"="TestMode/TestList") -> ("String Array"=w356:string[])  [unwired: 9 in, 1 out]
        n222 = Build Array (concatenate)("Select the test to run...", w356) -> (w355:string[])
        n223 = property on="Test Name" class="Ring (strict)"("Strings []"=w355) -> ()  [unwired: 2 in, 2 out]
      }
      event "Test Name": Value Change {
        w358 = FALSE ("Visible")
        # "Tell the robot the test name to run"
        n224 = event-data() -> ("NewVal"=w362:u16)  [unwired: 1 in]
        n225 = property on="Test Name" class="Ring (strict)"() -> ("Strings []"=w363:string[])  [unwired: 2 in, 2 out]
        n226 = local write "Progress"(T6 {"Test Progress"=0, "Test Progress Text"=""} ("Progress")) -> ()
        n227 = Index Array(array=w363, index=w362) -> (element=w361:string)
        n228 = call <vilib>:"NT Write String.vi"("String"=w361, "Name"="TestMode/TestName") -> ()  [unwired: 9 in, 1 out]
        n229 = property on="Progress" class="Clust (strict)"("Visible"=TRUE) -> ()  [unwired: 2 in, 2 out]
        n230 = property on="Motor" class="Clust (strict)"("Visible"=w358) -> ()  [unwired: 2 in, 2 out]
        n231 = property on="Test Slider" class="Slide (strict)"("Visible"=w358) -> ()  [unwired: 2 in, 2 out]
        n232 = property on="On/Off" class="Bool (strict)"("Visible"=w358) -> ()  [unwired: 2 in, 2 out]
        n233 = property on="Rev/Fwd" class="Clust (strict)"("Visible"=w358) -> ()  [unwired: 2 in, 2 out]
        n234 = property on="Test Ring" class="Ring (strict)"("Visible"=w358) -> ()  [unwired: 2 in, 2 out]
      }
      event "Select Auto": Mouse Enter {
        # "Populate the combo box with the list of autonomous options"
        n235 = event-data() -> ()  [unwired: 1 in, 1 out]
        n236 = call <vilib>:"NT Read String Array.vi"("Name"="Auto List") -> ("String Array"=w365:string[])  [unwired: 9 in, 1 out]
        n237 = property on="Select Auto" class="CmbBox"("Strings[]"=w365) -> ()  [unwired: 2 in, 2 out]
      }
      event "Select Auto": Value Change {
        # "User modified the Auto Selection. Write to NT variable so robot knows."
        n238 = event-data() -> ("NewVal"=w368:string)  [unwired: 1 in]
        n239 = call <vilib>:"NT Write String.vi"("String"=w368, "Name"="Auto Selector") -> ()  [unwired: 9 in, 1 out]
      }
      event "Command Selection": Value Change {
        # "Get the params and show in table"
        n240 = event-data() -> ("NewVal"=w374:i32)  [unwired: 1 in]
        n241 = property on="Command Selection" class="MCListbox (strict)"() -> ("ItemNames"=w372:string[][])  [unwired: 2 in, 2 out]
        n242 = call <vilib>:"WPI_DashboardUpdate Command Params.vi"("NewVal"=w374, "Commands"=w372, "Param Tbl"=w373) -> ()  [unwired: 8 in, 1 out]
      }
      event "Execute Command": Value Change {
        # "Started one, Unique ID holds\nresponse"
        n243 = event-data() -> ()  [unwired: 1 in, 1 out]
        n244 = property on="Command Selection" class="MCListbox (strict)"() -> ("ItemNames"=w385:string[][])  [unwired: 2 in, 2 out]
        n245 = Index Array(array=w385, index (row)="Command Selection", index (col)=0) -> (element=w383:string)
        n246 = call <vilib>:"Invoke Commands.vi"("Command Params"="Command Params", "Function Name"=w383) -> ("Params"=w379:u8, "Started"=w378:bool)  [unwired: 7 in, 1 out]
        n247 = Array Subset(array="Command Params", length (row)=w379) -> (w380:string[][])  [unwired: 3 in]
        n248 = Select(t="Executing" ("Cmd Status"), s=w378, f="" ("Cmd Status")) -> (s? t:f=→"Cmd Status":string)
      }
      event "Command Selection": Double Click {
        n249 = event-data() -> ("Row"=w393:i32)  [unwired: 1 in]
        n250 = property on="Command Selection" class="MCListbox (strict)"() -> ("ItemNames"=w396:string[][])  [unwired: 2 in, 2 out]
        n251 = local read "Command Params"() -> (w392:string[][])
        n252 = Index Array(array=w396, index (row)=w393, index (col)=0) -> (element=w394:string)
        n253 = call <vilib>:"Invoke Commands.vi"("Command Params"=w392, "Function Name"=w394) -> ("Params"=w391:u8, "Started"=w386:bool)  [unwired: 7 in, 1 out]
        n254 = Array Subset(array=w392, length (row)=w391) -> (w390:string[][])  [unwired: 3 in]
        n255 = Select(t="Executing" ("Cmd Status"), s=w386, f="" ("Cmd Status")) -> (s? t:f=w387:string)
        n256 = local write "Cmd Status"(w387) -> ()
      }
      event "CheckList": Double Click {
        # "Shift clears all"
        # "Update symbols on the listbox"
        n257 = event-data() -> ("PlatMods.Shift"=w398:bool, "Row"=w400:i32)  [unwired: 1 in]
        n258 = case shown="True" w398 {
          tunnel: w400 -> [w404 _]
          tunnel: 1 -> [w403 _]
          frame False {
            n259 = property on="CheckList" class="LstBox (strict)"() -> ("Item Symbols"=w402:i32[])  [unwired: 2 in, 2 out]
            n260 = Replace Array Subset(array=w402, new element=w403, index=w404) -> (w401:i32[])
            n261 = property on="CheckList" class="LstBox (strict)"("Item Symbols"=w401) -> ()  [unwired: 2 in, 2 out]
          }
          frame True {
            w405 = 0 ("Top Row")
            n262 = property on="CheckList" class="LstBox (strict)"() -> ("Number of Rows"=w407:u32)  [unwired: 2 in, 2 out]
            n263 = Initialize Array(0, w407) -> (w406:i32[])
            n264 = property on="CheckList" class="LstBox (strict)"("Top Row"=w405, "Value"=w405, "Item Symbols"=w406) -> ()  [unwired: 2 in, 2 out]
          }
        }
      }
      event "CheckList": Key Down {
        # "Update symbols on the listbox\nLeft and right keys check and uncheck"
        n265 = event-data() -> ("VKey"=w411:T20)  [unwired: 1 in]
        n266 = case shown="\"Left\", \"Right\"" w411 {
          selector: w411 -> [w416 _]
          tunnel: eventvkey."Left" ("VKey") -> [w414 _]
          frame "Left", "Right" {
            n267 = Equal?(x=w414, y=w416) -> (x = y?=w415:bool)
            n268 = Select(t=0, s=w415, f=1) -> (s? t:f=w417:i32)
            n269 = property on="CheckList" class="LstBox (strict)"() -> ("Item Symbols"=w420:i32[])  [unwired: 2 in, 2 out]
            n270 = Replace Array Subset(array=w420, new element=w417, index="CheckList") -> (w419:i32[])
            n271 = property on="CheckList" class="LstBox (strict)"("Item Symbols"=w419) -> ()  [unwired: 2 in, 2 out]
          }
          frame Default {
          }
        }
      }
      event "Motor.Enable": Value Change {
        # "When the test mode otor enable helper is set, update that\ntree row item's value"
        n272 = event-data() -> ("NewVal"=w426:bool)  [unwired: 1 in]
        n273 = Unbundle("Motor") -> ("Value"=w425:dbl)  [unwired: 1 out]
        n274 = Select(t=w425, s=w426, f=0.0) -> (s? t:f=w423:dbl)
        n275 = call <vilib>:"NT Write Number.vi"("Numeric"=w423, "Name"=w422) -> ()  [unwired: 9 in, 1 out]
      }
      event "Test Slider": Value Change {
        # "When the test mode slider helper is set, update that\ntree row item's value"
        n276 = event-data() -> ("NewVal"=w429:dbl)  [unwired: 1 in]
        n277 = call <vilib>:"NT Write Number.vi"("Numeric"=w429, "Name"=w430) -> ()  [unwired: 9 in, 1 out]
      }
      event "On/Off": Value Change {
        # "When the test mode on/off helper value is set, update that\ntree row item's value"
        n278 = event-data() -> ("NewVal"=w434:bool)  [unwired: 1 in]
        n279 = Boolean To (0,1)(Boolean=w434) -> (0, 1=w433:i16)
        n280 = call <vilib>:"NT Write Number.vi"("Numeric"=w433, "Name"=w432) -> ()  [unwired: 9 in, 1 out]
      }
      event "Rev/Fwd": Value Change {
        # "When the test mode helper value for relays is set, update that\ntree row item's value"
        n281 = event-data() -> ("NewVal.Forward"=w442:bool, "NewVal.Reverse"=w441:bool)  [unwired: 1 in]
        n282 = Boolean To (0,1)(Boolean=w442) -> (0, 1=w438:i16)
        n283 = Boolean To (0,1)(Boolean=w441) -> (0, 1=w440:i16)
        n284 = Negate(x=w440) -> (-x=w439:i16)
        n285 = Add(x=w438, y=w439) -> (x+y=w437:i16)
        n286 = call <vilib>:"NT Write Number.vi"("Numeric"=w437, "Name"=w436) -> ()  [unwired: 9 in, 1 out]
      }
      event "Test Ring": Value Change {
        # "When a test mode helper value is selected from the ring,\nset the tree item's variable to the string value"
        n287 = event-data() -> ("NewVal"=w446:u16)  [unwired: 1 in]
        n288 = property on="Test Ring" class="Ring (strict)"() -> ("Strings []"=w447:string[])  [unwired: 2 in, 2 out]
        n289 = Index Array(array=w447, index=w446) -> (element=w445:string)
        n290 = call <vilib>:"NT Write String.vi"("String"=w445, "Name"=w444) -> ()  [unwired: 9 in, 1 out]
      }
      event "Rec Mode": Value Change {
        # "Update globals for recording mode and path to read log from.\nClear when logging and let NetworkTables set path for vision to\nuse."
        n291 = event-data() -> ("NewVal"=w458:enum32{"Stop", "Record", "Playback"})  [unwired: 1 in]
        n292 = global write "WPI_DashboardLogging Global.vi" "Logging Filename"(path "") -> ()
        n293 = global write "WPI_DashboardLogging Global.vi" "Recording"(w458) -> ()
        n294 = case shown="\"Playback\"" w458 {
          tunnel: w457 -> [_ w460 w469]
          tunnel: [_ _ w468] -> w455
          tunnel: [_ _ w467] -> _
          tunnel: w453 -> [_ _ w465]
          tunnel: cluster{i32, i32} {-250, 170} -> [_ _ w464]
          tunnel: [_ _ T21 {"Image Size"=TRUE, "Image Type"=TRUE, "Pixel Value"=TRUE, "ROI Information"=TRUE, "Zoom Factor"=FALSE} ("Image Information Shown:All Elements")] -> w448
          tunnel: [_ _ TRUE ("Zoom Factor")] -> w449
          tunnel: w451 -> [_ _ w461]
          frame Default {
          }
          frame "Stop", "Record" {
            # "Place Window too"
            n295 = invoke class="VI" method="FP.Close"(reference=w460) -> (reference out=w459:refnum<vi>)  [unwired: 2 in, 2 out]
            n296 = invoke class="VI" method="Abort VI"(reference=w459) -> ()  [unwired: 2 in, 3 out]
          }
          frame "Playback" {
            n297 = call "Open Playback Panel.vi"("Offset"=w464, "DB VI Ref"=w465, "Playback in"=w469) -> ("Playback out"=w466:refnum<vi>)  [unwired: 8 in]
            n298 = register-events(w466, w461) -> (reference out=w468:refnum<event-registration>, error out=w467:errorcluster)  [unwired: 2 in]
          }
        }
        n299 = property on="Camera Image Right" class="ImageControl"("Image Information Shown"=w448, "Image Information Visible"=w449) -> ()  [unwired: 2 in, 2 out]
        n300 = property on="Camera Image" class="ImageControl"("Image Information Shown"=w448, "Image Information Visible"=w449) -> ()  [unwired: 2 in, 2 out]
        n301 = call <vilib>:"WPI_DashboardNT Log FieldName Cache.vi"("Operation"=enum16{"Lookup/Add", "Index", "Clear"}."Clear") -> ()  [unwired: 8 in, 3 out]
      }
      event Panel Close {
        w471 = enum32{"Stop", "Record", "Playback"}."Stop" ("Rec Mode")
        # "Playback window has been closed, abort"
        n302 = event-data() -> ()  [unwired: 1 in, 4 out]
        n303 = local write "Rec Mode"(w471) -> ()
        n304 = global write "WPI_DashboardLogging Global.vi" "Recording"(w471) -> ()
      }
      event Panel Close {
        # "Abort playback window and ourself"
        n305 = event-data() -> ()  [unwired: 1 in, 4 out]
        n306 = invoke class="VI" method="FP.Close"(reference=w475) -> (reference out=w474:refnum<vi>)  [unwired: 2 in, 2 out]
        n307 = invoke class="VI" method="Abort VI"(reference=w474) -> (error out=w473:errorcluster)  [unwired: 2 in, 2 out]
        n308 = invoke class="VI" method="Abort VI"(error in=w473) -> ()  [unwired: 2 in, 3 out]
      }
      event User Event {
        n309 = event-data() -> ("IDs"=w482:cluster{"RPC field ID":u16, "Unique ID":u16}, "String"=w481:string)  [unwired: 1 in]
        n310 = Bundle("IDs"=w482, "String"=w481) -> (w480:T9)  [unwired: 1 in]
        n311 = call <vilib>:"Retrieve RPC Response.vi"("RPC Response"=w480) -> ("Output"=w478:string[][])  [unwired: 10 in]
        n312 = Build Array (concatenate)(w476, w478) -> (w477:string[][])
        n313 = local write "Command Params"(w477) -> ()
        n314 = local write "Cmd Status"("" ("Cmd Status")) -> ()
      }
      event "Tree": Double Click {
        n315 = event-data() -> ("PlatMods"=w488:T24, "Tag"=w485:string)  [unwired: 1 in]
        n316 = Unbundle(w488) -> ("Shift"=w487:bool)  [unwired: 4 out]
        n317 = String Subset(string=w485, length (rest)=1 ("length (rest)")) -> (substring=w484:string)  [unwired: 1 in]
        n318 = Not(x=w487) -> (.not. x?=w486:bool)
        n319 = case shown="\"/\"" w484 {
          tunnel: w485 -> [_ w491]
          tunnel: w486 -> [_ w490]
          frame Default {
          }
          frame "/" {
            n320 = call <vilib>:"NT Update Persistence.vi"("Persistence"=w490, "Name"=w491) -> ()  [unwired: 9 in, 1 out]
          }
        }
      }
    }
  }
  n321 = while {
    tunnel: w65 -> [w493]
    i -> [w496]
    stop <- FALSE stop-if-true
    n322 = Wait (ms)(milliseconds to wait=u32 100) -> ()  [unwired: 1 out]
    n323 = case shown="\"Playback\"" "Rec Mode" {
      tunnel: w496 -> [_ _ w511]
      tunnel: [u32 2829099 ("Base Color") u32 11141120 ("Target Color") w500] -> w492
      frame "Stop", Default {
        # "Reset the color, extra updates don't cost much"
      }
      frame "Record" {
      }
      frame "Playback" {
        # "Playback"
        n324 = Quotient & Remainder(x=w511, y=u32 50 ("milliseconds to wait")) -> (x-y*floor(x/y)=w507:u32)  [unwired: 1 out]
        n325 = Divide(x=w507, y=u32 50 ("milliseconds to wait")) -> (x/y=w504:dbl)
        n326 = Multiply(x=6.283185307179586, y=w504) -> (x*y=w509:dbl)
        n327 = Sine(x=w509) -> (sin(x)=w508:dbl)
        n328 = Absolute Value(x=w508) -> (abs(x)=w501:dbl)
        n329 = call "Interpolate RGB Color.vi"("Proportion"=w501, "Target Color"=u32 30976, "Base Color"=u32 2829099) -> ("Result Color"=w500:u32)  [unwired: 8 in]
      }
    }
    n330 = property class="Pane"(reference=w493, "PaneColor"=w492) -> ()  [unwired: 1 in, 2 out]
  }
  n331 = local write "Dashboard Tab"(T2."Drive" ("Dashboard Tab")) -> ()
  n332 = property on="On/Off" class="Bool (strict)"("Visible"=w36) -> ()  [unwired: 2 in, 2 out]
  n333 = property on="Motor" class="Clust (strict)"("Visible"=w36) -> ()  [unwired: 2 in, 2 out]
  n334 = property on="Progress" class="Clust (strict)"("Visible"=w36) -> ()  [unwired: 2 in, 2 out]
  n335 = property on="Test Ring" class="Ring (strict)"("Visible"=w36) -> ()  [unwired: 2 in, 2 out]
  n336 = property on="Rev/Fwd" class="Clust (strict)"("Visible"=w36) -> ()  [unwired: 2 in, 2 out]
  n337 = while {
    tunnel: u16 1741 ("timeout ms (25000)") -> [w513]
    stop <- FALSE stop-if-true
    n338 = TCP Create Listener(10:w513) -> (0:w512:errorcluster, 3:w514:refnum<k5>)  [unwired: 4 in, 1 out]
    n339 = case shown="No Error" w512 {
      selector: w512 -> [w516 _]
      tunnel: w514 -> [w517 _]
      frame No Error {
        n340 = while {
          tunnel: w517 -> [w520]
          tunnel: w516 -> [w519]
          stop <- FALSE stop-if-true
          n341 = TCP Wait On Listener(8:w519, 11:w520) -> (0:w521:errorcluster, 4:w522:refnum<k5>)  [unwired: 2 in, 3 out]
          n342 = local write "TCP"(w522) -> ()
          n343 = case shown="No Error" w521 {
            frame No Error {
            }
            frame Error {
              n344 = Wait (ms)(milliseconds to wait=u32 1000) -> ()  [unwired: 1 out]
            }
          }
        }
      }
      frame Error {
        n345 = Wait (ms)(milliseconds to wait=u32 1000) -> ()  [unwired: 1 out]
      }
    }
  }
  n346 = local write "Command Selection"(u16 0 ("milliseconds to wait")) -> ()
  n347 = local write "Command Params"(string[][] [] ("Command Params")) -> ()
  n348 = global write "WPI_DashboardLogging Global.vi" "Recording"(w59) -> ()
  n349 = local write "Rec Mode"(w59) -> ()
  n350 = call <vilib>:"NT Write String.vi"("String"="Select Auto", "Name"="Auto Selector") -> ()  [unwired: 9 in, 1 out]
